vi "Server Side.vi"() -> ()   [LabVIEW 2021]
panel:
  in  "Stop":bool
  in  "Floating Menu":T1(tab)
  in  "Curtains":T2 {"Kitchen 3" scale=0.0..10.0; "Kitchen 2" scale=0.0..10.0; "Kitchen 1" scale=0.0..10.0; "Living Room" scale=0.0..10.0; "Bedroom 2-B" scale=0.0..10.0; "Bedroom 1-B" scale=0.0..10.0; "Master Bedroom" scale=0.0..10.0; "Bedroom 2-A" scale=0.0..10.0; "Bedroom 1-A" scale=0.0..10.0}
  in  "Lights":T3
  in  "Doors":T4
  in  "TV":T5 {"Volume" scale=0.0..100.0}
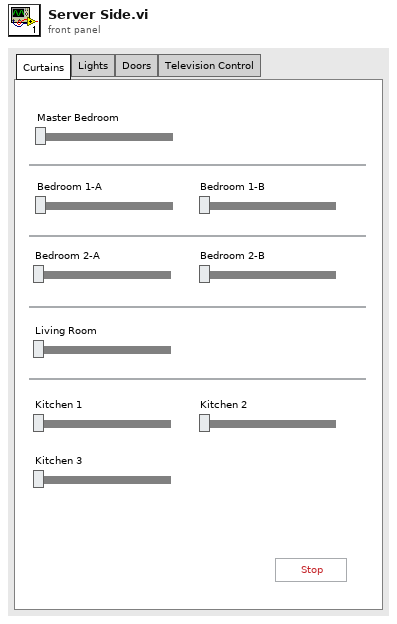
[diagram p1: front panel]
types:
  T1 = enum32{"Curtains", "Lights", "Doors", "Television Control"}
  T2 = cluster{"Master Bedroom":dbl, "Bedroom 1-A":dbl, "Bedroom 1-B":dbl, "Bedroom 2-A":dbl, "Bedroom 2-B":dbl, "Living Room":dbl, "Kitchen 1":dbl, "Kitchen 2":dbl, "Kitchen 3":dbl}
  T3 = cluster{"M Bedroom 1":bool, "M Bedroom 2":bool, "Bedroom 1":bool, "Bedroom 2":bool, "L Room 1":bool, "L Room 2":bool, "Kitchen":bool, "L Room Toilet":bool, "Kitchen Toilet":bool, "Kitchen Toilet 2":bool, "Balcony 1":bool, "Balcony 2":bool, "Balcony 3":bool}
  T4 = cluster{"M Room-L Room":bool, "M Room-Toilet":bool, "M Room-Balcony":bool, "Bedroom 1-L Room":bool, "Bedroom 2-L Room":bool, "L Room Balcony":bool, "L Room":bool, "Kitchen-Balcony":bool, "L Room-Toilet":bool, "Living Room-Kitchen":bool, "Kitchen-Toilet 2":bool, "B1-A":bool, "B1-B":bool, "B1-C":bool, "B2-A":bool, "B2-B":bool, "B2-C":bool, "MB-A":bool, "MB-B":bool, "MB-C":bool}
  T5 = cluster{"Seek Back Button":bool, "Seek Forward Button":bool, "Remove Button":bool, "Add Button":bool, "Stop Button":bool, "Volume":dbl}
  T6 = cluster{"Curtains":cluster{"Master Bedroom":dbl, "Bedroom 1-A":dbl, "Bedroom 1-B":dbl, "Bedroom 2-A":dbl, "Bedroom 2-B":dbl, "Living Room":dbl, "Kitchen 1":dbl, "Kitchen 2":dbl, "Kitchen 3":dbl}, "Lights":cluster{"M Bedroom 1":bool, "M Bedroom 2":bool, "Bedroom 1":bool, "Bedroom 2":bool, "L Room 1":bool, "L Room 2":bool, "Kitchen":bool, "L Room Toilet":bool, "Kitchen Toilet":bool, "Kitchen Toilet 2":bool, "Balcony 1":bool, "Balcony 2":bool, "Balcony 3":bool}, "Doors":cluster{"M Room-L Room":bool, "M Room-Toilet":bool, "M Room-Balcony":bool, "Bedroom 1-L Room":bool, "Bedroom 2-L Room":bool, "L Room Balcony":bool, "L Room":bool, "Kitchen-Balcony":bool, "L Room-Toilet":bool, "Living Room-Kitchen":bool, "Kitchen-Toilet 2":bool, "B1-A":bool, "B1-B":bool, "B1-C":bool, "B2-A":bool, "B2-B":bool, "B2-C":bool, "MB-A":bool, "MB-B":bool, "MB-C":bool}, "TV":cluster{"Seek Back Button":bool, "Seek Forward Button":bool, "Remove Button":bool, "Add Button":bool, "Stop Button":bool, "Volume":dbl}}
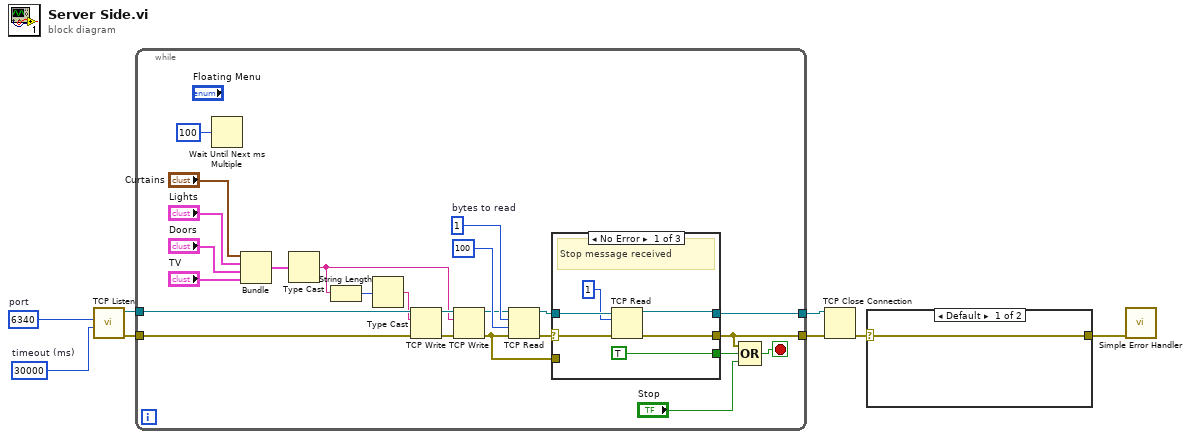
[diagram p0: block diagram]
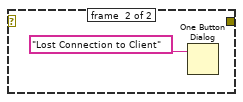
[diagram p4: hidden frame]
diagram:
  w7 = u16 6340  # port
  w8 = 30000  # timeout (ms)
  n1 = call <vilib>:"TCP Listen.vi"("timeout ms (wait forever: -1)"=w8, "port"=w7) -> ("error out"=w5:errorcluster, "connection ID"=w6:refnum<k5>)  [unwired: 5 in, 3 out]
  n2 = while {
    tunnel: w5 -> [w31]
    tunnel: [w28] -> w1
    tunnel: w6 -> [w32]
    tunnel: [w30] -> w2
    stop <- w29 stop-if-true
    w22 = 1  # bytes to read
    n3 = Wait Until Next ms Multiple(millisecond multiple=u32 100) -> ()  [unwired: 1 out]
    n4 = Bundle("Curtains"="Curtains", "Lights"="Lights", "Doors"="Doors", "TV"="TV") -> (w11:T6)  [unwired: 1 in]
    n5 = Type Cast(x=w11) -> (*(type *) &x=w23:string)  [unwired: 1 out]
    n6 = String Length(string=w23) -> (length=w25:i32)
    n7 = Type Cast(x=w25) -> (*(type *) &x=w24:string)  [unwired: 1 out]
    n8 = TCP Write(connection ID=w32, data in=w24, error in (no error)=w31) -> (connection ID out=w27:refnum<k5>, error out=w26:errorcluster)  [unwired: 2 out]
    n9 = TCP Write(connection ID=w27, data in=w23, error in (no error)=w26) -> (connection ID out=w20:refnum<k5>, error out=w19:errorcluster)  [unwired: 2 out]
    n10 = TCP Read(connection ID=w20, bytes to read=w22, error in (no error)=w19, 9:100 ("milliseconds to wait")) -> (connection ID out=w17:refnum<k5>, error out=w18:errorcluster)  [unwired: 2 out]
    n11 = case shown="No Error" w18 {
      selector: w18 -> [w35 _ w42]
      tunnel: [w33 w40 w42] -> w28
      tunnel: w19 -> [_ w40 _]
      tunnel: [TRUE _ _] -> w16
      tunnel: w17 -> [w37 w39 w41]
      tunnel: [w36 w39 w41] -> w30
      frame No Error {
        # "Stop message received"
        n12 = TCP Read(connection ID=w37, bytes to read=1, error in (no error)=w35) -> (connection ID out=w36:refnum<k5>, error out=w33:errorcluster)  [unwired: 1 in, 2 out]
      }
      frame Error {
        # "Timed out; no stop message received"
      }
      frame Default {
        # "Some other error occurred"
      }
    }
    n13 = Compound Arithmetic op=OR(w28, w16, "Stop") -> (w29:bool)
  }
  n14 = TCP Close Connection(connection ID=w2, error in (no error)=w1) -> (error out=w4:errorcluster)  [unwired: 2 out]
  n15 = case shown="Default" w4 {
    selector: w4 -> [w43 _]
    tunnel: [w43 _] -> w3
    frame #0 {
    }
    frame #1 {
      n16 = One Button Dialog(message="Lost Connection to Client" ("Client Closed")) -> ()  [unwired: 1 in, 1 out]
    }
  }
  n17 = call <vilib>:"Simple Error Handler.vi"("error in (no error)"=w3) -> ()  [unwired: 1 in, 8 out]
